vi "Update Motors.vi"(0 "VFD Refs":refnum<vi>[](array[refnum]), 1 "PLC Coils":bool[](array[boolean]), 2 "PLC Regs":u16[](array[numeric]), 3 "Motor Data IN":T1(array[cluster])) -> (14 "Motor Data OUT":T1(array[cluster]))   [LabVIEW 2020]
uses:
  Type Defs/Motor Type Type Def.ctl
  Type Defs/PLC Coils.ctl
  Type Defs/PLC Registers.ctl
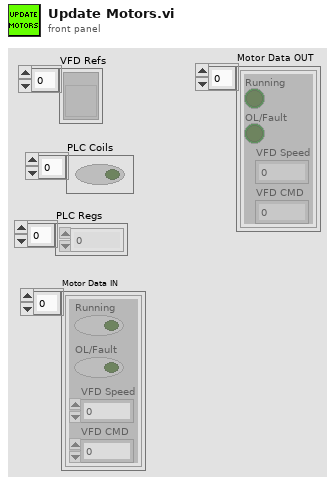
[diagram p1: front panel]
types:
  T1 = cluster{"Running":bool, "OL/Fault":bool, "VFD Speed":dbl, "VFD CMD":dbl}[]
  T2 = typedef "Motor Type Type Def.ctl" = enum16{"MS", "VFD"}
  T3 = typedef "PLC Coils.ctl" = enum16{"MC200_PLC_Estop_Main", "MC201_PLC_Estop_GSI", "MC202_PLC_Estop_Dryer", "MC203_PLC_Auto_Mode", "MC204", "MC205", "MC206", "MC207", "MC208", "MC209", "MC210", "MC211", "MC212", "MC213", "MC214", "MC215", "MC216", "MC217", "MC218", "MC219", "MC220_PLC_WS_Drag_ON", "MC221_PLC_WB_Drag_ON", "MC222_PLC_WS_Fan_ON", "MC223_PLC_WB_Fan_ON", "MC224_PLC_Dryr_Drag_ON", "MC225_PLC_Dryr_Fan_ON", "MC226", "MC227", "MC228", "MC229", "MC230", "MC231", "MC232", "MC233", "MC234", "MC235", "MC236", "MC237", "MC238", "MC239", "MC240_PLC_WS_Drag_OL", "MC241_PLC_WB_Drag_OL", "MC242_PLC_WS_Fan_OL", "MC243_PLC_WB_Fan_OL", "MC244_PLC_Dryr_Drag_OL", "MC245_PLC_Dryr_Fan_OL", "MC246_PLC_DB_Fan_Alm", "MC247_PLC_DB_Drag_Alm", "MC248_PLC_DB_Tp_Fd_Alm", "MC249_PLC_U_Trough_Alm", "MC250_PLC_Leg_Alm", "MC251", "MC252", "MC253", "MC254", "MC255", "MC256", "MC257", "MC258", "MC259", "MC260_PLC_Dryer_Full", "MC261_PLC_Dryer_HI_Alm", "MC262_PLC_Dryr_Bin_Full", "MC263_PLC_DB_HI_Alm", "MC264_PLC_Dryer_Chute", "MC265_PLC_Dryer_Feed", "MC266", "MC267", "MC268", "MC269", "MC270_PLC_WS_Limit", "MC271_PLC_WB_Limit", "MC272_PLC_Dryr_Bin_Lim", "MC273_PLC_DB_Limit", "MC274_PLC_Auto_Leg_Dry", "MC275", "MC276", "MC277", "MC278", "MC279", "MC280_Auto_Error_0", "MC281_Auto_Error_1", "MC282_Auto_Error_2", "MC283_Auto_Error_3", "MC284_Auto_Error_4", "MC285_Auto_Error_5", "MC286_Auto_Error_6", "MC287_Auto_Error_7", "MC288_Auto_Error_8", "MC289_Auto_Error_9"}
  T4 = typedef "PLC Registers.ctl" = enum16{"MHR200_PLC_DB_Fan_Spd", "MHR201_PLC_DB_Drag_Spd", "MHR202_PLC_DB_Tp_Fd_Spd", "MHR203_PLC_U_Trough_Spd", "MHR204_PLC_Leg_Spd", "MHR205_PLC_DB_Fan_ON", "MHR206_PLC_DB_Drag_ON", "MHR207_PLC_DB_Tp_Fd_ON", "MHR208_PLC_U_Trough_ON", "MHR209_PLC_Leg_ON", "MHR210_PLC_DB_Fan_CMD", "MHR211_PLC_DB_Drag_CMD", "MHR212_PLC_DB_Tp_Fd_CMD", "MHR213_PLC_U_Trough_CMD", "MHR214_PLC_Leg_CMD", "MHR215_PLC_DB_Fan_Flt", "MHR216_PLC_DB_Drag_Flt", "MHR217_PLC_DB_Tp_Fd_Flt", "MHR218_PLC_U_Trough_Flt", "MHR219_PLC_Leg_Flt", "MHR220_PLC_DB_Level", "MHR221_PLC_WB_Level", "MHR222_PLC_WS_Level", "MHR223_PLC_Dryr_Bin_Level", "MHR224_PLC_Leg_Amps", "MHR225_PLC_DB_Tp_Fd_Amps"}
  T5 = cluster{"Running":bool, "OL/Fault":bool, "VFD Speed":dbl, "VFD CMD":dbl}
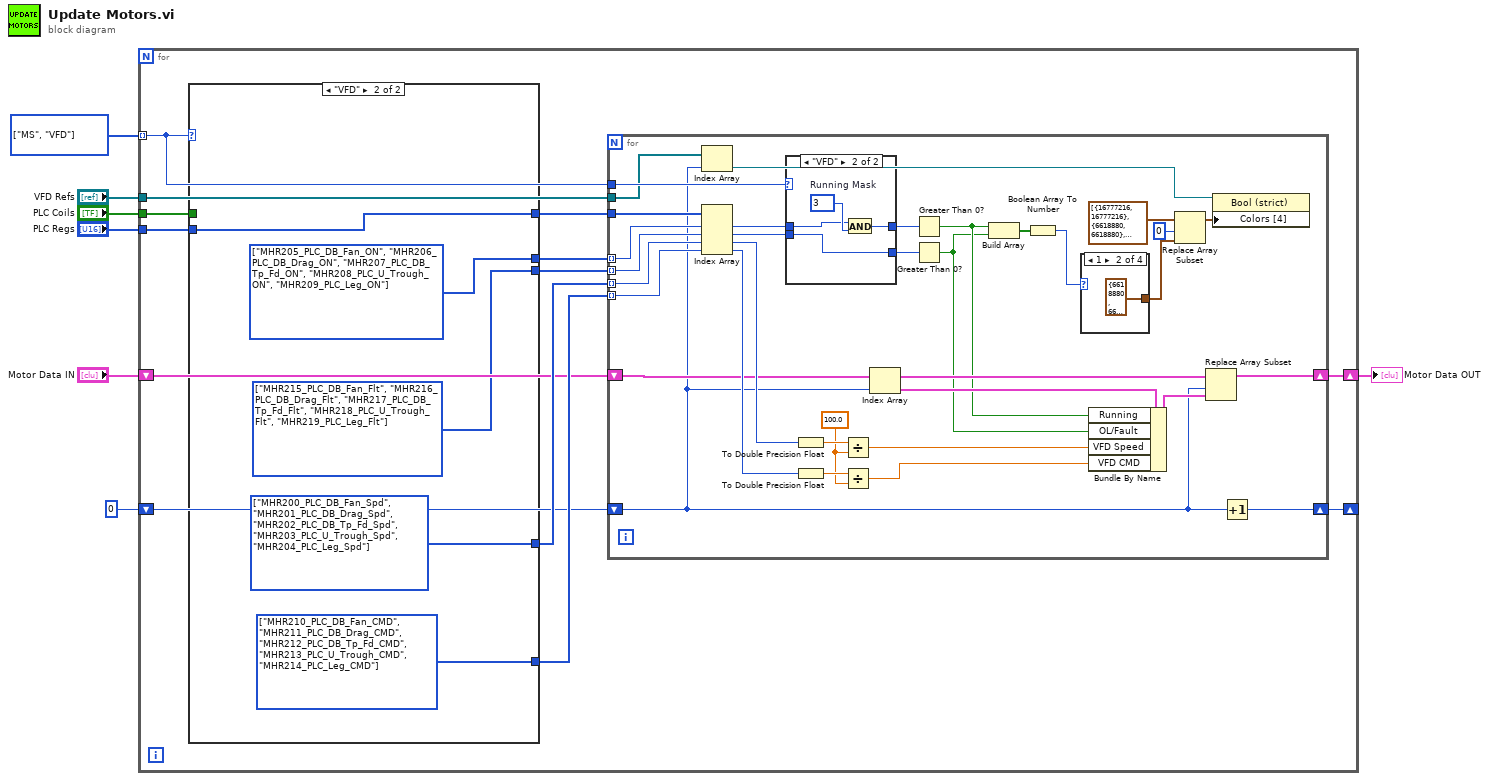
[diagram p0: block diagram]
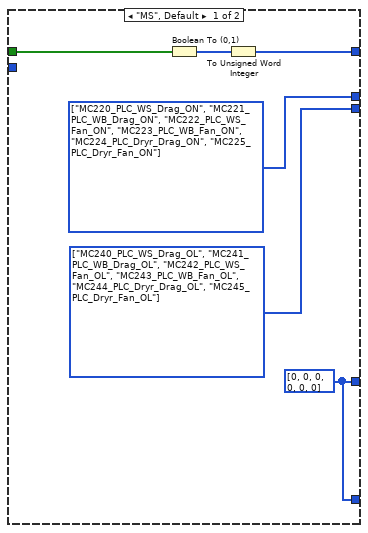
[diagram p2: hidden frame]
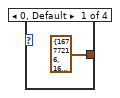
[diagram p4: hidden frame]
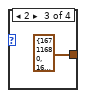
[diagram p5: hidden frame]
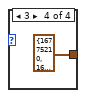
[diagram p6: hidden frame]
diagram:
  w4 = T2[] [enum."MS", enum."VFD"] items=["MS", "VFD"]
  n1 = for {
    tunnel: "PLC Regs" -> [w18]
    tunnel: "PLC Coils" -> [w16]
    tunnel: "VFD Refs" -> [w14]
    tunnel: w4 -> [w15] mode=indexing
    shift-right: [w10] -> w2
    shift-left: "Motor Data IN" -> [w11]
    shift-right: [w8] -> _
    shift-left: 0 ("index") -> [w9]
    n2 = case shown="\"VFD\"" w15 {
      tunnel: [w26 w29] -> w20
      tunnel: [w25 w30] -> w19
      tunnel: [w22 w31] -> w17
      tunnel: w18 -> [_ w31]
      tunnel: w16 -> [w24 _]
      tunnel: [w21 w28] -> w13
      tunnel: [w21 w27] -> w12
      frame "MS", Default {
        w21 = u16[] [0, 0, 0, 0, 0, 0] ("PLC Regs")
        w26 = T3[] [enum."MC240_PLC_WS_Drag_OL", enum."MC241_PLC_WB_Drag_OL", enum."MC242_PLC_WS_Fan_OL", enum."MC243_PLC_WB_Fan_OL", enum."MC244_PLC_Dryr_Drag_OL", enum."MC245_PLC_Dryr_Fan_OL"] items=["MC200_PLC_Estop_Main", "MC201_PLC_Estop_GSI", "MC202_PLC_Estop_Dryer", "MC203_PLC_Auto_Mode", "MC204", "MC205", "MC206", "MC207", "MC208", "MC209", "MC210", "MC211", "MC212", "MC213", "MC214", "MC215", "MC216", "MC217", "MC218", "MC219", "MC220_PLC_WS_Drag_ON", "MC221_PLC_WB_Drag_ON", "MC222_PLC_WS_Fan_ON", "MC223_PLC_WB_Fan_ON", "MC224_PLC_Dryr_Drag_ON", "MC225_PLC_Dryr_Fan_ON", "MC226", "MC227", "MC228", "MC229", "MC230", "MC231", "MC232", "MC233", "MC234", "MC235", "MC236", "MC237", "MC238", "MC239", "MC240_PLC_WS_Drag_OL", "MC241_PLC_WB_Drag_OL", "MC242_PLC_WS_Fan_OL", "MC243_PLC_WB_Fan_OL", "MC244_PLC_Dryr_Drag_OL", "MC245_PLC_Dryr_Fan_OL", "MC246_PLC_DB_Fan_Alm", "MC247_PLC_DB_Drag_Alm", "MC248_PLC_DB_Tp_Fd_Alm", "MC249_PLC_U_Trough_Alm", "MC250_PLC_Leg_Alm", "MC251", "MC252", "MC253", "MC254", "MC255", "MC256", "MC257", "MC258", "MC259", "MC260_PLC_Dryer_Full", "MC261_PLC_Dryer_HI_Alm", "MC262_PLC_Dryr_Bin_Full", "MC263_PLC_DB_HI_Alm", "MC264_PLC_Dryer_Chute", "MC265_PLC_Dryer_Feed", "MC266", "MC267", "MC268", "MC269", "MC270_PLC_WS_Limit", "MC271_PLC_WB_Limit", "MC272_PLC_Dryr_Bin_Lim", "MC273_PLC_DB_Limit", "MC274_PLC_Auto_Leg_Dry", "MC275", "MC276", "MC277", "MC278", "MC279", "MC280_Auto_Error_0", "MC281_Auto_Error_1", "MC282_Auto_Error_2", "MC283_Auto_Error_3", "MC284_Auto_Error_4", "MC285_Auto_Error_5", "MC286_Auto_Error_6", "MC287_Auto_Error_7", "MC288_Auto_Error_8", "MC289_Auto_Error_9"]
        w25 = T3[] [enum."MC220_PLC_WS_Drag_ON", enum."MC221_PLC_WB_Drag_ON", enum."MC222_PLC_WS_Fan_ON", enum."MC223_PLC_WB_Fan_ON", enum."MC224_PLC_Dryr_Drag_ON", enum."MC225_PLC_Dryr_Fan_ON"] items=["MC200_PLC_Estop_Main", "MC201_PLC_Estop_GSI", "MC202_PLC_Estop_Dryer", "MC203_PLC_Auto_Mode", "MC204", "MC205", "MC206", "MC207", "MC208", "MC209", "MC210", "MC211", "MC212", "MC213", "MC214", "MC215", "MC216", "MC217", "MC218", "MC219", "MC220_PLC_WS_Drag_ON", "MC221_PLC_WB_Drag_ON", "MC222_PLC_WS_Fan_ON", "MC223_PLC_WB_Fan_ON", "MC224_PLC_Dryr_Drag_ON", "MC225_PLC_Dryr_Fan_ON", "MC226", "MC227", "MC228", "MC229", "MC230", "MC231", "MC232", "MC233", "MC234", "MC235", "MC236", "MC237", "MC238", "MC239", "MC240_PLC_WS_Drag_OL", "MC241_PLC_WB_Drag_OL", "MC242_PLC_WS_Fan_OL", "MC243_PLC_WB_Fan_OL", "MC244_PLC_Dryr_Drag_OL", "MC245_PLC_Dryr_Fan_OL", "MC246_PLC_DB_Fan_Alm", "MC247_PLC_DB_Drag_Alm", "MC248_PLC_DB_Tp_Fd_Alm", "MC249_PLC_U_Trough_Alm", "MC250_PLC_Leg_Alm", "MC251", "MC252", "MC253", "MC254", "MC255", "MC256", "MC257", "MC258", "MC259", "MC260_PLC_Dryer_Full", "MC261_PLC_Dryer_HI_Alm", "MC262_PLC_Dryr_Bin_Full", "MC263_PLC_DB_HI_Alm", "MC264_PLC_Dryer_Chute", "MC265_PLC_Dryer_Feed", "MC266", "MC267", "MC268", "MC269", "MC270_PLC_WS_Limit", "MC271_PLC_WB_Limit", "MC272_PLC_Dryr_Bin_Lim", "MC273_PLC_DB_Limit", "MC274_PLC_Auto_Leg_Dry", "MC275", "MC276", "MC277", "MC278", "MC279", "MC280_Auto_Error_0", "MC281_Auto_Error_1", "MC282_Auto_Error_2", "MC283_Auto_Error_3", "MC284_Auto_Error_4", "MC285_Auto_Error_5", "MC286_Auto_Error_6", "MC287_Auto_Error_7", "MC288_Auto_Error_8", "MC289_Auto_Error_9"]
        n3 = Boolean To (0,1)(Boolean=w24) -> (0, 1=w23:i16[])
        n4 = To Unsigned Word Integer(number=w23) -> (unsigned 16bit integer=w22:u16[])
      }
      frame "VFD" {
        w27 = T4[] [enum."MHR210_PLC_DB_Fan_CMD", enum."MHR211_PLC_DB_Drag_CMD", enum."MHR212_PLC_DB_Tp_Fd_CMD", enum."MHR213_PLC_U_Trough_CMD", enum."MHR214_PLC_Leg_CMD"] items=["MHR200_PLC_DB_Fan_Spd", "MHR201_PLC_DB_Drag_Spd", "MHR202_PLC_DB_Tp_Fd_Spd", "MHR203_PLC_U_Trough_Spd", "MHR204_PLC_Leg_Spd", "MHR205_PLC_DB_Fan_ON", "MHR206_PLC_DB_Drag_ON", "MHR207_PLC_DB_Tp_Fd_ON", "MHR208_PLC_U_Trough_ON", "MHR209_PLC_Leg_ON", "MHR210_PLC_DB_Fan_CMD", "MHR211_PLC_DB_Drag_CMD", "MHR212_PLC_DB_Tp_Fd_CMD", "MHR213_PLC_U_Trough_CMD", "MHR214_PLC_Leg_CMD", "MHR215_PLC_DB_Fan_Flt", "MHR216_PLC_DB_Drag_Flt", "MHR217_PLC_DB_Tp_Fd_Flt", "MHR218_PLC_U_Trough_Flt", "MHR219_PLC_Leg_Flt", "MHR220_PLC_DB_Level", "MHR221_PLC_WB_Level", "MHR222_PLC_WS_Level", "MHR223_PLC_Dryr_Bin_Level", "MHR224_PLC_Leg_Amps", "MHR225_PLC_DB_Tp_Fd_Amps"]
        w28 = T4[] [enum."MHR200_PLC_DB_Fan_Spd", enum."MHR201_PLC_DB_Drag_Spd", enum."MHR202_PLC_DB_Tp_Fd_Spd", enum."MHR203_PLC_U_Trough_Spd", enum."MHR204_PLC_Leg_Spd"] items=["MHR200_PLC_DB_Fan_Spd", "MHR201_PLC_DB_Drag_Spd", "MHR202_PLC_DB_Tp_Fd_Spd", "MHR203_PLC_U_Trough_Spd", "MHR204_PLC_Leg_Spd", "MHR205_PLC_DB_Fan_ON", "MHR206_PLC_DB_Drag_ON", "MHR207_PLC_DB_Tp_Fd_ON", "MHR208_PLC_U_Trough_ON", "MHR209_PLC_Leg_ON", "MHR210_PLC_DB_Fan_CMD", "MHR211_PLC_DB_Drag_CMD", "MHR212_PLC_DB_Tp_Fd_CMD", "MHR213_PLC_U_Trough_CMD", "MHR214_PLC_Leg_CMD", "MHR215_PLC_DB_Fan_Flt", "MHR216_PLC_DB_Drag_Flt", "MHR217_PLC_DB_Tp_Fd_Flt", "MHR218_PLC_U_Trough_Flt", "MHR219_PLC_Leg_Flt", "MHR220_PLC_DB_Level", "MHR221_PLC_WB_Level", "MHR222_PLC_WS_Level", "MHR223_PLC_Dryr_Bin_Level", "MHR224_PLC_Leg_Amps", "MHR225_PLC_DB_Tp_Fd_Amps"]
        w29 = T4[] [enum."MHR215_PLC_DB_Fan_Flt", enum."MHR216_PLC_DB_Drag_Flt", enum."MHR217_PLC_DB_Tp_Fd_Flt", enum."MHR218_PLC_U_Trough_Flt", enum."MHR219_PLC_Leg_Flt"] items=["MHR200_PLC_DB_Fan_Spd", "MHR201_PLC_DB_Drag_Spd", "MHR202_PLC_DB_Tp_Fd_Spd", "MHR203_PLC_U_Trough_Spd", "MHR204_PLC_Leg_Spd", "MHR205_PLC_DB_Fan_ON", "MHR206_PLC_DB_Drag_ON", "MHR207_PLC_DB_Tp_Fd_ON", "MHR208_PLC_U_Trough_ON", "MHR209_PLC_Leg_ON", "MHR210_PLC_DB_Fan_CMD", "MHR211_PLC_DB_Drag_CMD", "MHR212_PLC_DB_Tp_Fd_CMD", "MHR213_PLC_U_Trough_CMD", "MHR214_PLC_Leg_CMD", "MHR215_PLC_DB_Fan_Flt", "MHR216_PLC_DB_Drag_Flt", "MHR217_PLC_DB_Tp_Fd_Flt", "MHR218_PLC_U_Trough_Flt", "MHR219_PLC_Leg_Flt", "MHR220_PLC_DB_Level", "MHR221_PLC_WB_Level", "MHR222_PLC_WS_Level", "MHR223_PLC_Dryr_Bin_Level", "MHR224_PLC_Leg_Amps", "MHR225_PLC_DB_Tp_Fd_Amps"]
        w30 = T4[] [enum."MHR205_PLC_DB_Fan_ON", enum."MHR206_PLC_DB_Drag_ON", enum."MHR207_PLC_DB_Tp_Fd_ON", enum."MHR208_PLC_U_Trough_ON", enum."MHR209_PLC_Leg_ON"] items=["MHR200_PLC_DB_Fan_Spd", "MHR201_PLC_DB_Drag_Spd", "MHR202_PLC_DB_Tp_Fd_Spd", "MHR203_PLC_U_Trough_Spd", "MHR204_PLC_Leg_Spd", "MHR205_PLC_DB_Fan_ON", "MHR206_PLC_DB_Drag_ON", "MHR207_PLC_DB_Tp_Fd_ON", "MHR208_PLC_U_Trough_ON", "MHR209_PLC_Leg_ON", "MHR210_PLC_DB_Fan_CMD", "MHR211_PLC_DB_Drag_CMD", "MHR212_PLC_DB_Tp_Fd_CMD", "MHR213_PLC_U_Trough_CMD", "MHR214_PLC_Leg_CMD", "MHR215_PLC_DB_Fan_Flt", "MHR216_PLC_DB_Drag_Flt", "MHR217_PLC_DB_Tp_Fd_Flt", "MHR218_PLC_U_Trough_Flt", "MHR219_PLC_Leg_Flt", "MHR220_PLC_DB_Level", "MHR221_PLC_WB_Level", "MHR222_PLC_WS_Level", "MHR223_PLC_Dryr_Bin_Level", "MHR224_PLC_Leg_Amps", "MHR225_PLC_DB_Tp_Fd_Amps"]
      }
    }
    n5 = for {
      tunnel: w17 -> [w60]
      tunnel: w19 -> [w64] mode=indexing
      tunnel: w14 -> [w34]
      tunnel: w20 -> [w59] mode=indexing
      tunnel: w15 -> [w55]
      tunnel: w13 -> [w50] mode=indexing
      tunnel: w12 -> [w49] mode=indexing
      shift-right: [w43] -> w10
      shift-left: w11 -> [w42]
      shift-right: [w35] -> w8
      shift-left: w9 -> [w33]
      w45 = 100.0 ("y")
      n6 = Index Array(array=w34, index=w33) -> (element=w32:refnum<vi>)
      n7 = Index Array(array=w60, index #1=w64, index #2=w59, index #3=w50, index #4=w49) -> (element #1=w54:u16, element #2=w53:u16, element #3=w48:u16, element #4=w44:u16)
      n8 = case shown="\"VFD\"" w55 {
        tunnel: w54 -> [w66 w69]
        tunnel: w53 -> [w65 w67]
        tunnel: [w66 w68] -> w52
        tunnel: [w65 w67] -> w51
        frame "MS", Default {
        }
        frame "VFD" {
          w70 = u16 3  # Running Mask
          n9 = And(x=w69, y=w70) -> (x .and. y?=w68:u16)
        }
      }
      n10 = To Double Precision Float(number=w48) -> (double precision float=w47:dbl)
      n11 = To Double Precision Float(number=w44) -> (double precision float=w46:dbl)
      n12 = Divide(x=w47, y=w45) -> (x/y=w37:dbl)
      n13 = Divide(x=w46, y=w45) -> (x/y=w36:dbl)
      n14 = Index Array(array=w42, index=w33) -> (element=w41:T5)
      n15 = Greater Than 0?(x=w52) -> (x > 0?=w39:bool)
      n16 = Greater Than 0?(x=w51) -> (x > 0?=w38:bool)
      n17 = Build Array(w39, w38) -> (w58:bool[])
      n18 = Boolean Array To Number(Boolean array=w58) -> (number=w57:u32)
      n19 = case shown="1" w57 {
        tunnel: [cluster{u32, u32} {16777216, 16777216} cluster{u32, u32} {6618880, 6618880} cluster{u32, u32} {16711680, 16711680} cluster{u32, u32} {16775210, 16775210}] -> w56
        frame 0, Default {
        }
        frame 1 {
        }
        frame 2 {
        }
        frame 3 {
        }
      }
      n20 = Bundle By Name(cluster=w41, "Running"=w39, "OL/Fault"=w38, "VFD Speed"=w37, "VFD CMD"=w36) -> (w40:T5)
      n21 = Replace Array Subset(array=cluster{u32, u32}[] [{16777216, 16777216}, {6618880, 6618880}, {16777216, 16777216}, {3309312, 3309312}] ("Colors [4]"), new element=w56, index=0) -> (w61:cluster{u32, u32}[])
      n22 = Replace Array Subset(array=w42, new element=w40, index=w33) -> (w43:T1)
      n23 = property class="Bool (strict)"(reference=w32, "Colors [4]"=w61) -> ()  [unwired: 1 in, 2 out]
      n24 = Increment(x=w33) -> (x+1=w35:i32)
    }
  }
  "Motor Data OUT" <- w2
